vi "Native POST File Upload Example.vi"() -> ()   [LabVIEW 2017]
uses:
  <vilib>/httpClient/POSTFile.vi
  <vilib>/httpClient/LabVIEWHTTPClient.lvlib
panel:
  out "body":string
  out "headers":string
  in  "Authentication":cluster{"Username":string, "Password":string}
  out "error out":errorcluster
  in  "FIlepath":path=path "D:/upwork/Labview-REST-API/labview-source/payload.png"
  in  "API Endpoint Url":string="https://luferau.free.beeceptor.com/upload"
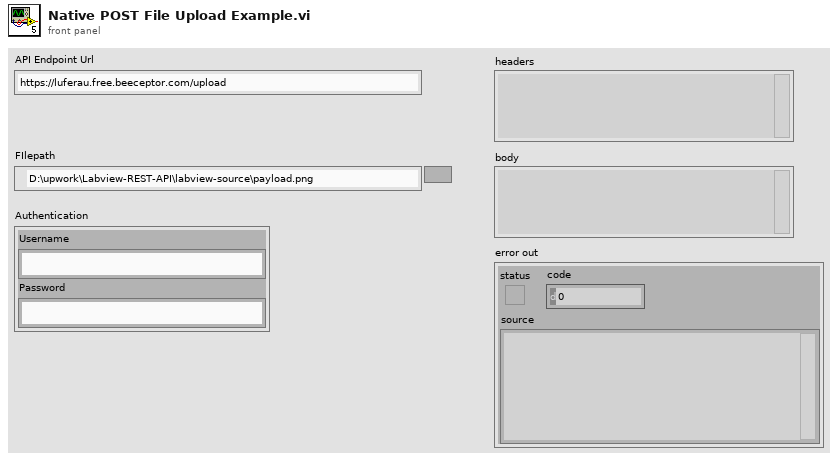
[diagram p1: front panel]
types:
  T1 = typedef "LabVIEWHTTPClient.lvlib/ClientHandle.ctl" = refnum<k1>
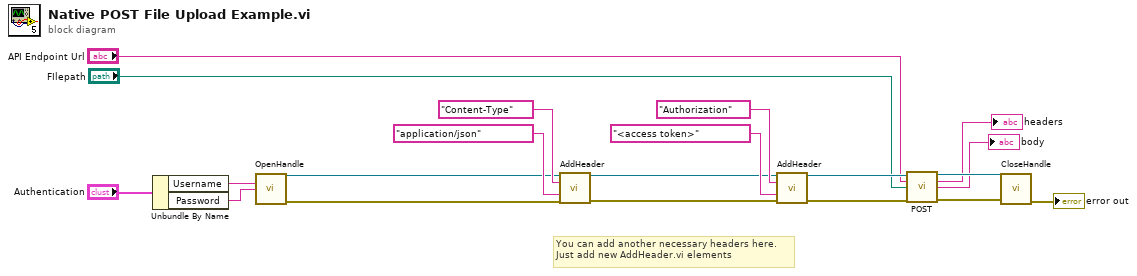
[diagram p0: block diagram]
diagram:
  # "You can add another necessary headers here.\nJust add new AddHeader.vi elements"
  n1 = Unbundle By Name("Authentication") -> ("Username"=w19:string, "Password"=w18:string)
  n2 = call <vilib>:"OpenHandle.vi"("username"=w19, "password"=w18) -> ("client handle out"=w1:T1, "error out"=w4:errorcluster)  [unwired: 12 in]
  n3 = call <vilib>:"AddHeader.vi"("client handle"=w1, "header"="Content-Type", "value"="application/json", "error in (no error)"=w4) -> ("client handle out"=w2:T1, "error out"=w3:errorcluster)  [unwired: 10 in]
  n4 = call <vilib>:"AddHeader.vi"("client handle"=w2, "header"="Authorization", "value"="<access token>", "error in (no error)"=w3) -> ("client handle out"=w14:T1, "error out"=w11:errorcluster)  [unwired: 10 in]
  n5 = call-poly <vilib>:"POST.vi"("client handle"=w14, "url"="API Endpoint Url", "file"="FIlepath", "error in (no error)"=w11) -> ("client handle out"=w10:T1, "headers"=→"headers":string, "body"=→"body":string, "error out"=w9:errorcluster)  [unwired: 8 in]
  n6 = call <vilib>:"CloseHandle.vi"("client handle"=w10, "error in (no error)"=w9) -> ("error out"=→"error out":errorcluster)  [unwired: 13 in]
